vi "RTInitializer (1).vi"() -> (0 "error out":errorcluster)   [LabVIEW 2017]
doc: "Ensures all outputs and variables are set to a safe value (FALSE for most), prior to running the rest of the VI. If values cannot be set for any reason, an error will be given, after a 10 second timeout."
uses:
  RTControl/ControlActivateSolenoidsGlobal.vi
  RTControl/StopGLOBAL.vi
  <vilib>/NI_Real-Time Target Support.lvlib
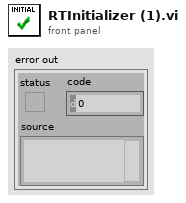
[diagram p1: front panel]
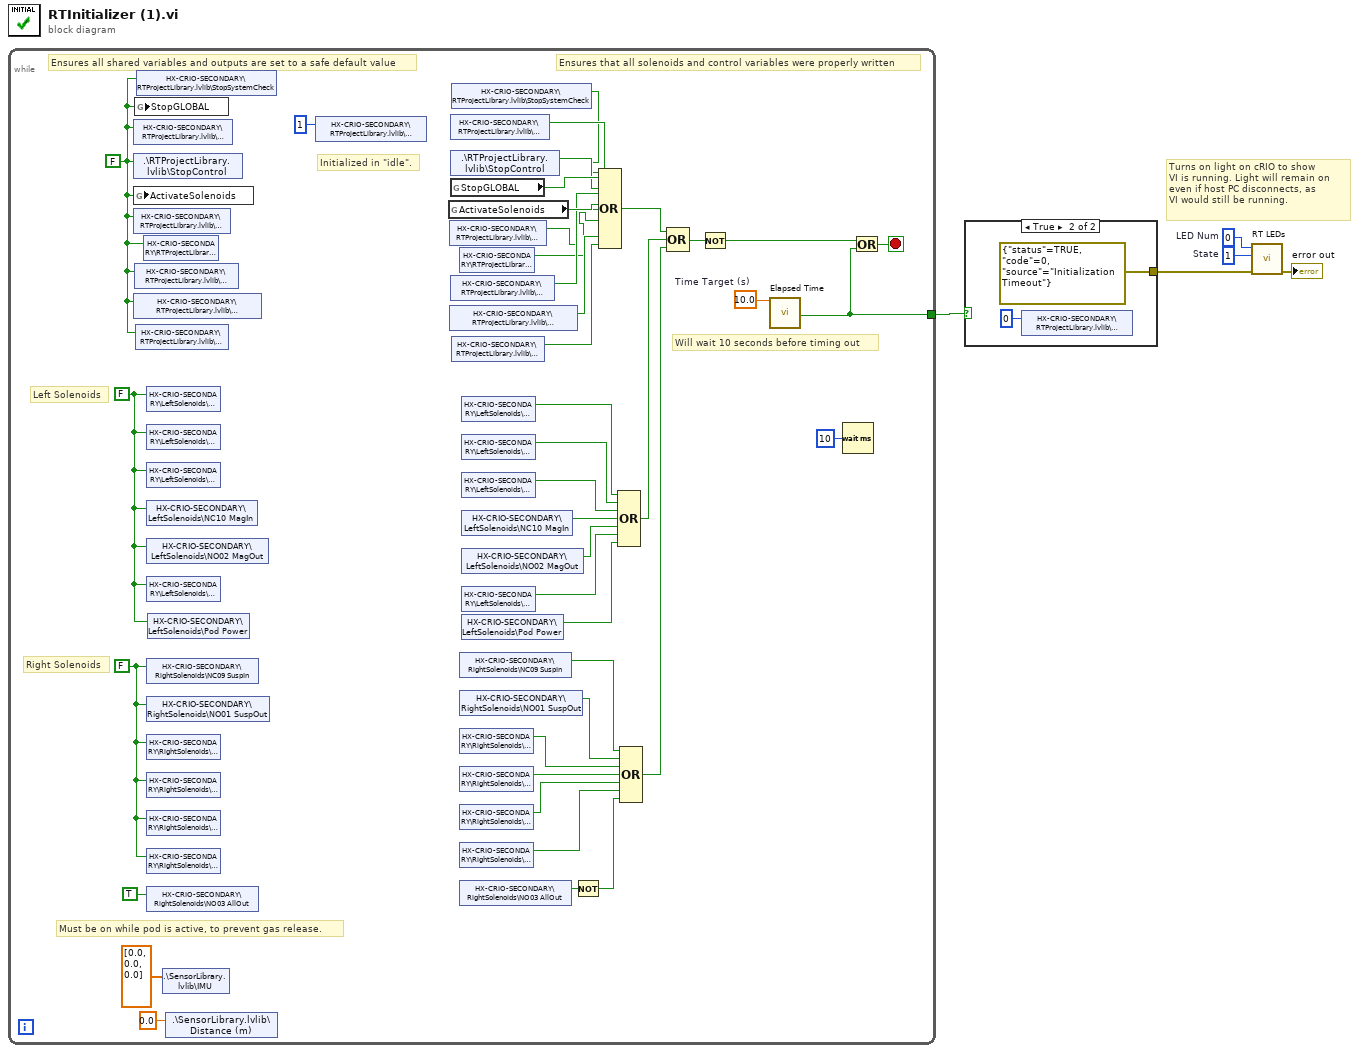
[diagram p0: block diagram]
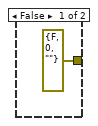
[diagram p2: hidden frame]
diagram:
  w2 = 0  # LED Num
  w3 = 1  # State
  # "Turns on light on cRIO to show\nVI is running. Light will remain on \neven if host PC disconnects, as \nVI would still be running."
  n1 = while {
    tunnel: [w41] -> w5
    stop <- w44 stop-if-true
    w43 = 10.0  # Time Target (s)
    w38 = FALSE ("NC03")
    w46 = FALSE ("NC09")
    w6 = FALSE ("Stop Control")
    # "Initialized in \"idle\"."
    # "Must be on while pod is active, to prevent gas release."
    # "Will wait 10 seconds before timing out"
    # "Ensures that all solenoids and control variables were properly written"
    # "Ensures all shared variables and outputs are set to a safe default value"
    # "Left Solenoids"
    # "Right Solenoids"
    n2 = shared-variable "HX-CRIO-SECONDARY\\RTProjectLibrary.lvlib\\PodPower"(w6) -> ()  [unwired: 1 in, 1 out]
    n3 = shared-variable ".\\RTProjectLibrary.lvlib\\StopControl"(w6) -> ()  [unwired: 1 in, 1 out]
    n4 = global write "ControlActivateSolenoidsGlobal.vi" "ActivateSolenoids"(w6) -> ()
    n5 = shared-variable "HX-CRIO-SECONDARY\\RTProjectLibrary.lvlib\\ClearError"(w6) -> ()  [unwired: 1 in, 1 out]
    n6 = shared-variable "HX-CRIO-SECONDARY\\RTProjectLibrary.lvlib\\EnableForceIdle"(w6) -> ()  [unwired: 1 in, 1 out]
    n7 = global write "StopGLOBAL.vi" "StopGLOBAL"(w6) -> ()
    n8 = shared-variable "HX-CRIO-SECONDARY\\RTProjectLibrary.lvlib\\Emergency"(w6) -> ()  [unwired: 1 in, 1 out]
    n9 = shared-variable "HX-CRIO-SECONDARY\\RTProjectLibrary.lvlib\\ForceIdle"(w6) -> ()  [unwired: 1 in, 1 out]
    n10 = shared-variable "HX-CRIO-SECONDARY\\RTProjectLibrary.lvlib\\StopSystemCheck"(w6) -> ()  [unwired: 1 in, 1 out]
    n11 = shared-variable "HX-CRIO-SECONDARY\\RTProjectLibrary.lvlib\\Abort"(w6) -> ()  [unwired: 1 in, 1 out]
    n12 = shared-variable "HX-CRIO-SECONDARY\\LeftSolenoids\\NC03"(w38) -> ()  [unwired: 1 in, 1 out]
    n13 = shared-variable "HX-CRIO-SECONDARY\\LeftSolenoids\\NC04"(w38) -> ()  [unwired: 1 in, 1 out]
    n14 = shared-variable "HX-CRIO-SECONDARY\\LeftSolenoids\\NC02"(w38) -> ()  [unwired: 1 in, 1 out]
    n15 = shared-variable "HX-CRIO-SECONDARY\\LeftSolenoids\\NC10 MagIn"(w38) -> ()  [unwired: 1 in, 1 out]
    n16 = shared-variable "HX-CRIO-SECONDARY\\LeftSolenoids\\NO02 MagOut"(w38) -> ()  [unwired: 1 in, 1 out]
    n17 = shared-variable "HX-CRIO-SECONDARY\\LeftSolenoids\\NC01"(w38) -> ()  [unwired: 1 in, 1 out]
    n18 = shared-variable "HX-CRIO-SECONDARY\\RightSolenoids\\NC09 SuspIn"(w46) -> ()  [unwired: 1 in, 1 out]
    n19 = shared-variable "HX-CRIO-SECONDARY\\RightSolenoids\\NO01 SuspOut"(w46) -> ()  [unwired: 1 in, 1 out]
    n20 = shared-variable "HX-CRIO-SECONDARY\\RightSolenoids\\NC08"(w46) -> ()  [unwired: 1 in, 1 out]
    n21 = shared-variable "HX-CRIO-SECONDARY\\RightSolenoids\\NC05"(w46) -> ()  [unwired: 1 in, 1 out]
    n22 = shared-variable "HX-CRIO-SECONDARY\\RightSolenoids\\NC06"(w46) -> ()  [unwired: 1 in, 1 out]
    n23 = shared-variable "HX-CRIO-SECONDARY\\RightSolenoids\\NC07"(w46) -> ()  [unwired: 1 in, 1 out]
    n24 = shared-variable "HX-CRIO-SECONDARY\\RightSolenoids\\NO03 AllOut"(TRUE ("NO03")) -> ()  [unwired: 1 in, 1 out]
    n25 = shared-variable "HX-CRIO-SECONDARY\\LeftSolenoids\\Pod Power"(w38) -> ()  [unwired: 1 in, 1 out]
    n26 = shared-variable ".\\SensorLibrary.lvlib\\IMU"(dbl[] [0.0, 0.0, 0.0] ("IMU")) -> ()  [unwired: 1 in, 1 out]
    n27 = shared-variable ".\\SensorLibrary.lvlib\\Distance (m)"(0.0 ("Distance (m)")) -> ()  [unwired: 1 in, 1 out]
    n28 = shared-variable "HX-CRIO-SECONDARY\\RTProjectLibrary.lvlib\\CurrentState"(u8 1 ("CurrentState")) -> ()  [unwired: 1 in, 1 out]
    n29 = global read "ControlActivateSolenoidsGlobal.vi" "ActivateSolenoids"() -> (w36:bool)
    n30 = shared-variable "HX-CRIO-SECONDARY\\RTProjectLibrary.lvlib\\ClearError"() -> (w10:bool)  [unwired: 1 in, 1 out]
    n31 = shared-variable "HX-CRIO-SECONDARY\\RTProjectLibrary.lvlib\\EnableForceIdle"() -> (w13:bool)  [unwired: 1 in, 1 out]
    n32 = shared-variable "HX-CRIO-SECONDARY\\RTProjectLibrary.lvlib\\PodPower"() -> (w33:bool)  [unwired: 1 in, 1 out]
    n33 = shared-variable ".\\RTProjectLibrary.lvlib\\StopControl"() -> (w34:bool)  [unwired: 1 in, 1 out]
    n34 = global read "StopGLOBAL.vi" "StopGLOBAL"() -> (w35:bool)
    n35 = shared-variable "HX-CRIO-SECONDARY\\RTProjectLibrary.lvlib\\Emergency"() -> (w12:bool)  [unwired: 1 in, 1 out]
    n36 = shared-variable "HX-CRIO-SECONDARY\\RTProjectLibrary.lvlib\\StopSystemCheck"() -> (w7:bool)  [unwired: 1 in, 1 out]
    n37 = shared-variable "HX-CRIO-SECONDARY\\RTProjectLibrary.lvlib\\ForceIdle"() -> (w14:bool)  [unwired: 1 in, 1 out]
    n38 = shared-variable "HX-CRIO-SECONDARY\\RTProjectLibrary.lvlib\\Abort"() -> (w11:bool)  [unwired: 1 in, 1 out]
    n39 = shared-variable "HX-CRIO-SECONDARY\\RightSolenoids\\NC09 SuspIn"() -> (w19:bool)  [unwired: 1 in, 1 out]
    n40 = shared-variable "HX-CRIO-SECONDARY\\RightSolenoids\\NO01 SuspOut"() -> (w20:bool)  [unwired: 1 in, 1 out]
    n41 = shared-variable "HX-CRIO-SECONDARY\\RightSolenoids\\NC08"() -> (w21:bool)  [unwired: 1 in, 1 out]
    n42 = shared-variable "HX-CRIO-SECONDARY\\RightSolenoids\\NC05"() -> (w22:bool)  [unwired: 1 in, 1 out]
    n43 = shared-variable "HX-CRIO-SECONDARY\\RightSolenoids\\NC06"() -> (w23:bool)  [unwired: 1 in, 1 out]
    n44 = shared-variable "HX-CRIO-SECONDARY\\RightSolenoids\\NC07"() -> (w24:bool)  [unwired: 1 in, 1 out]
    n45 = shared-variable "HX-CRIO-SECONDARY\\RightSolenoids\\NO03 AllOut"() -> (w39:bool)  [unwired: 1 in, 1 out]
    n46 = shared-variable "HX-CRIO-SECONDARY\\LeftSolenoids\\NC03"() -> (w32:bool)  [unwired: 1 in, 1 out]
    n47 = shared-variable "HX-CRIO-SECONDARY\\LeftSolenoids\\NC04"() -> (w31:bool)  [unwired: 1 in, 1 out]
    n48 = shared-variable "HX-CRIO-SECONDARY\\LeftSolenoids\\NC02"() -> (w30:bool)  [unwired: 1 in, 1 out]
    n49 = shared-variable "HX-CRIO-SECONDARY\\LeftSolenoids\\NC10 MagIn"() -> (w29:bool)  [unwired: 1 in, 1 out]
    n50 = shared-variable "HX-CRIO-SECONDARY\\LeftSolenoids\\NO02 MagOut"() -> (w28:bool)  [unwired: 1 in, 1 out]
    n51 = shared-variable "HX-CRIO-SECONDARY\\LeftSolenoids\\NC01"() -> (w27:bool)  [unwired: 1 in, 1 out]
    n52 = shared-variable "HX-CRIO-SECONDARY\\LeftSolenoids\\Pod Power"() -> (w26:bool)  [unwired: 1 in, 1 out]
    n53 = Not(x=w39) -> (.not. x?=w25:bool)
    n54 = Compound Arithmetic op=OR(w7, w33, w34, w35, w36, w10, w11, w12, w13, w14) -> (w17:bool)
    n55 = Compound Arithmetic op=OR(w32, w31, w30, w29, w28, w27, w26) -> (w15:bool)
    n56 = Compound Arithmetic op=OR(w19, w20, w21, w22, w23, w24, w25) -> (w16:bool)
    n57 = Compound Arithmetic op=OR(w17, w15, w16) -> (w18:bool)
    n58 = Not(x=w18) -> (.not. x?=w45:bool)
    n59 = call "Elapsed Time"("Time Target (s)"=w43) -> ("Time has Elapsed"=w41:bool)  [unwired: 11 in, 7 out]
    n60 = Wait (ms)(milliseconds to wait=u32 10 ("millisecond multiple")) -> ()  [unwired: 1 out]
    n61 = Or(x=w45, y=w41) -> (x .or. y?=w44:bool)
  }
  n62 = case shown="True" w5 {
    tunnel: [errorcluster {"status"=FALSE, "code"=0, "source"=""} ("error out") errorcluster {"status"=TRUE, "code"=0, "source"="Initialization Timeout"} ("error out")] -> w4
    frame False {
    }
    frame True {
      n63 = shared-variable "HX-CRIO-SECONDARY\\RTProjectLibrary.lvlib\\CurrentState"(u8 0 ("CurrentState")) -> ()  [unwired: 1 in, 1 out]
    }
  }
  n64 = call <vilib>:"RT LEDs.vi"("error in (no error)"=w4, "State"=w3, "LED Num"=w2) -> ("error out"=→"error out":errorcluster)  [unwired: 3 in, 1 out]
